vi "sy,,etry.vi"(10 "Array 2":dbl[](array[numeric]), 11 "Array":dbl[](array[numeric])) -> (3 "x-y 3":dbl)   [LabVIEW 2020]
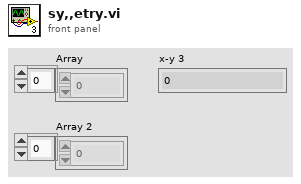
[diagram p1: front panel]
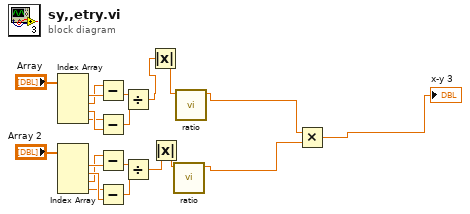
[diagram p0: block diagram]
diagram:
  n1 = Index Array(array="Array") -> (element #1=w15:dbl, element #2=w14:dbl, element #3=w17:dbl, element #4=w16:dbl)  [unwired: 4 in]
  n2 = Index Array(array="Array 2") -> (element #1=w10:dbl, element #2=w12:dbl, element #3=w9:dbl, element #4=w11:dbl)  [unwired: 4 in]
  n3 = Subtract(x=w14, y=w15) -> (x-y=w20:dbl)
  n4 = Subtract(x=w16, y=w17) -> (x-y=w21:dbl)
  n5 = Subtract(x=w9, y=w10) -> (x-y=w18:dbl)
  n6 = Subtract(x=w11, y=w12) -> (x-y=w19:dbl)
  n7 = Divide(x=w20, y=w21) -> (x/y=w4:dbl)
  n8 = Divide(x=w18, y=w19) -> (x/y=w2:dbl)
  n9 = Absolute Value(x=w4) -> (abs(x)=w3:dbl)
  n10 = Absolute Value(x=w2) -> (abs(x)=w1:dbl)
  n11 = call "ratio.vi"("Numeric in"=w1) -> ("Numeric out"=w6:dbl)  [unwired: 10 in]
  n12 = call "ratio.vi"("Numeric in"=w3) -> ("Numeric out"=w7:dbl)  [unwired: 10 in]
  n13 = Multiply(x=w7, y=w6) -> (x*y=→"x-y 3":dbl)
